vi "DAC_Test.vi"() -> ()   [LabVIEW 2012]
panel:
  in  "x":dbl
  in  "Channel":u16
  in  "DeviceIndex":u64
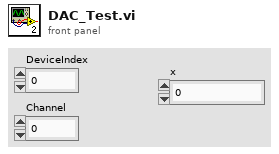
[diagram p1: front panel]
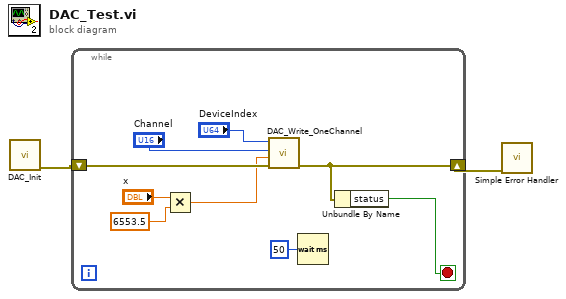
[diagram p0: block diagram]
diagram:
  n1 = call "DAC_Init.vi"() -> ("error out"=w1:errorcluster)  [unwired: 11 in]
  n2 = while {
    shift-right: [w8] -> w2
    shift-left: w1 -> [w9]
    stop <- w7 stop-if-true
    n3 = Multiply(x="x", y=6553.5) -> (x*y=w3:dbl)
    n4 = call "DAC_Write_OneChannel.vi"("error in (no error)"=w9, "Value"=w3, "Channel"="Channel", "DeviceIndex"="DeviceIndex") -> ("error out"=w8:errorcluster)  [unwired: 6 in, 1 out]
    n5 = Wait (ms)(milliseconds to wait=u32 50) -> ()  [unwired: 1 out]
    n6 = Unbundle By Name(w8) -> ("status"=w7:bool)
  }
  n7 = call <vilib>:"Simple Error Handler.vi"("error in (no error)"=w2) -> ()  [unwired: 4 in, 5 out]
